vi "knob driver 3.vi"() -> ()   [LabVIEW 2015]
uses:
  Stage/Move stage command.ctl
  h-nu-ixon/knob global.vi
panel:
  out "Device numbers":i32[](array[numeric])
  out "Encoder serial numbers":i32[](array[numeric])
  in  "um per turn":dbl[](array[numeric])=[10.0, 10.0, 1.0]
  out "Knob positions":i32[](array[knob]) scale=0.0..80.0
  in  "Quit":bool
  # "x\n\ny\n\nz"
  # "x\ny\nz"
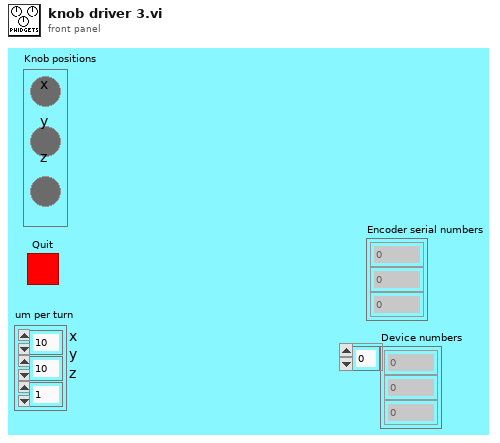
[diagram p1: front panel]
types:
  T1 = typedef "Move stage command.ctl" = cluster{"dx (um) (0 -> ignore)":ext, "dy (um) (0 -> ignore)":ext, "dz (um) (0 -> ignore)":ext, "Re-center x,y":bool, "Re-center z":bool, "x (um) (-1 -> ignore)":dbl, "y (um) (-1 -> ignore)":dbl, "z (um) (-1 -> ignore)":dbl}
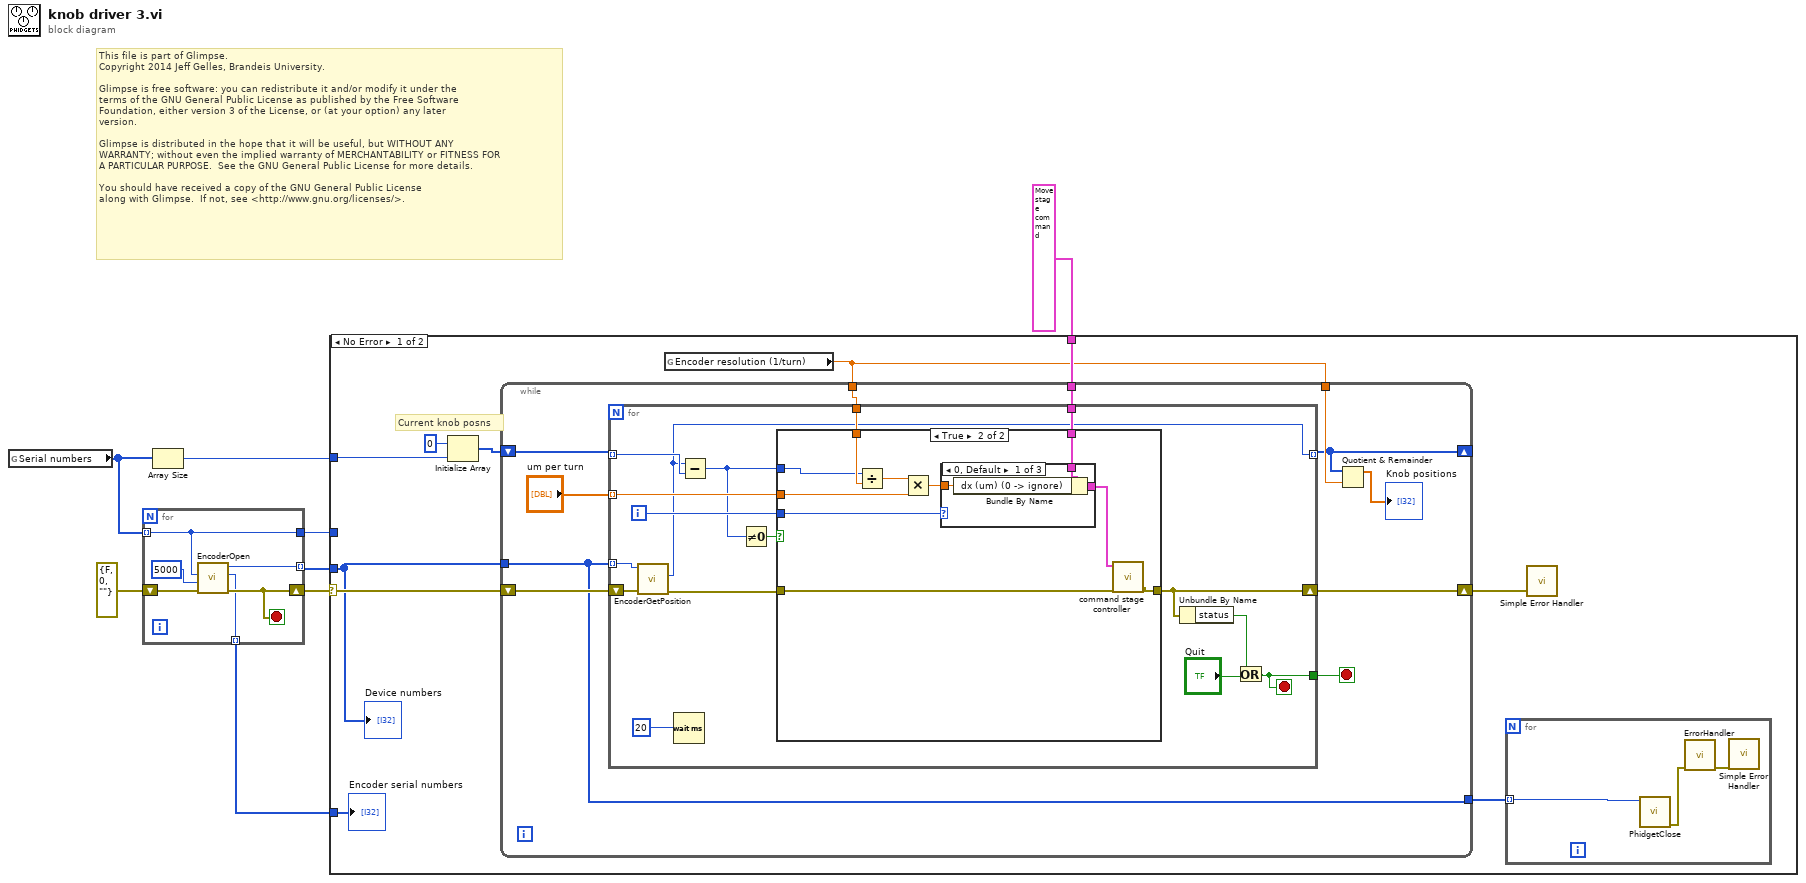
[diagram p0: block diagram]
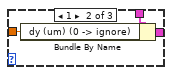
[diagram p3: hidden frame]
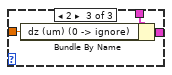
[diagram p4: hidden frame]
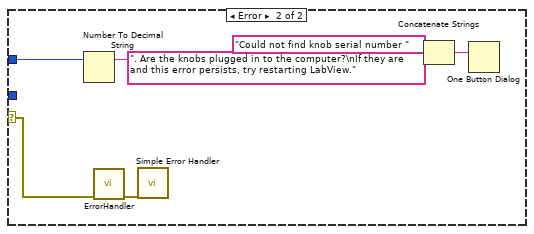
[diagram p5: hidden frame]
diagram:
  # "This file is part of Glimpse. \nCopyright 2014 Jeff Gelles, Brandeis University.    \n\nGlimpse is free software: you can redistribute it and/or modify it under the \nterms of the GNU General Public License as published by the Free Software \nFoundation, either version 3 of the License, or (at your option) any later \nversion.\n\nGlimpse is distributed in the hope that it will be useful, but WITHOUT ANY \nWARRANTY; without even the implied warranty of MERCHANTABILITY or FITNESS FOR \nA PARTICULAR PURPOSE.  See the GNU General Public License for more details.\n\nYou should have received a copy of the GNU General Public License\nalong with Glimpse.  If not, see <http://www.gnu.org/licenses/>."
  n1 = global read "knob global.vi" "Serial numbers"() -> (w4:i32[])
  n2 = for {
    tunnel: w4 -> [w11] mode=indexing
    shift-right: [w12] -> w7
    shift-left: errorcluster {"status"=FALSE, "code"=0, "source"=""} ("error in (no error)") -> [w14]
    tunnel: [w13] -> w5 mode=indexing
    tunnel: [w11] -> w6
    tunnel: [w10] -> w1 mode=indexing
    stop <- w12 stop-if-true
    n3 = call <userlib>:"EncoderOpen.vi"("error in (no error)"=w14, "milliseconds (5000)"=5000, "Serial Number (-1)"=w11) -> ("error out"=w12:errorcluster, "Serial Number Return"=w10:i32, "Device Out"=w13:i32)  [unwired: 5 in, 1 out]
  }
  n4 = Array Size(array=w4) -> (size(s)=w3:i32)
  n5 = case shown="No Error" w7 {
    selector: w7 -> [w16 w76]
    tunnel: w6 -> [_ w79]
    tunnel: w5 -> [w15 _]
    tunnel: w3 -> [w22 _]
    tunnel: T1 {"dx (um) (0 -> ignore)"=0.0, "dy (um) (0 -> ignore)"=0.0, "dz (um) (0 -> ignore)"=0.0, "Re-center x,y"=FALSE, "Re-center z"=FALSE, "x (um) (-1 -> ignore)"=-1.0, "y (um) (-1 -> ignore)"=-1.0, "z (um) (-1 -> ignore)"=-1.0} ("command") -> [w21 _]
    tunnel: w1 -> [w17 _]
    frame No Error {
      # "Current knob posns"
      n6 = Initialize Array(0 ("Position"), w22) -> (w24:i32[])
      n7 = global read "knob global.vi" "Encoder resolution (1/turn)"() -> (w20:dbl)
      n8 = while {
        shift-right: [w37] -> w19
        shift-left: w16 -> [w38]
        tunnel: w15 -> [w29]
        shift-right: [w30] -> _
        shift-left: w24 -> [w36]
        tunnel: w21 -> [w33]
        tunnel: w20 -> [w32]
        tunnel: w20 -> [w31]
        tunnel: [w29] -> w18
        stop <- w35 stop-if-true
        n9 = for {
          tunnel: w29 -> [w39] mode=indexing
          tunnel: [w47] -> w35
          shift-right: [w48] -> w37
          shift-left: w38 -> [w41]
          tunnel: [w44] -> w30 mode=indexing
          tunnel: w36 -> [w45] mode=indexing
          tunnel: "um per turn" -> [w54] mode=indexing
          tunnel: w33 -> [w53]
          tunnel: w32 -> [w51]
          i -> [w52]
          stop <- w47 stop-if-true
          n10 = call <userlib>:"EncoderGetPosition.vi"("error in (no error)"=w41, "Device In"=w39) -> ("error out"=w40:errorcluster, "Position"=w44:i32)  [unwired: 7 in, 1 out]
          n11 = Wait (ms)(milliseconds to wait=20) -> ()  [unwired: 1 out]
          n12 = Subtract(x=w44, y=w45) -> (x-y=w42:i32)
          n13 = Not Equal To 0?(x=w42) -> (x != 0?=w43:bool)
          n14 = case shown="True" w43 {
            tunnel: w54 -> [_ w65]
            tunnel: w53 -> [_ w64]
            tunnel: w52 -> [_ w63]
            tunnel: w51 -> [_ w62]
            tunnel: [w55 w61] -> w48
            tunnel: w40 -> [w55 w56]
            tunnel: w42 -> [_ w57]
            frame False {
            }
            frame True {
              n15 = Divide(x=w57, y=w62) -> (x/y=w58:dbl)
              n16 = Multiply(x=w58, y=w65) -> (x*y=w59:dbl)
              n17 = case shown="0, Default" w63 {
                tunnel: w64 -> [w68 w71 w74]
                tunnel: [w67 w70 w73] -> w60
                tunnel: w59 -> [w66 w69 w72]
                frame 0, Default {
                  n18 = Bundle By Name(cluster=w68, "dx (um) (0 -> ignore)"=w66) -> (w67:T1)
                }
                frame 1 {
                  n19 = Bundle By Name(cluster=w71, "dy (um) (0 -> ignore)"=w69) -> (w70:T1)
                }
                frame 2 {
                  n20 = Bundle By Name(cluster=w74, "dz (um) (0 -> ignore)"=w72) -> (w73:T1)
                }
              }
              n21 = call "command stage controller.vi"("command"=w60, "error in (no error)"=w56) -> ("error out"=w61:errorcluster)  [unwired: 6 in]
            }
          }
          n22 = Unbundle By Name(w48) -> ("status"=w49:bool)
          n23 = Or(x=w49, y="Quit") -> (x .or. y?=w47:bool)
        }
        n24 = Quotient & Remainder(x=w30, y=w31) -> (x-y*floor(x/y)=→"Knob positions":dbl[])  [unwired: 1 out]
      }
      n25 = for {
        tunnel: w18 -> [w25] mode=indexing
        n26 = call <userlib>:"PhidgetClose.vi"("Device In"=w25) -> ("error out"=w26:errorcluster)  [unwired: 10 in]
        n27 = call <userlib>:"ErrorHandler.vi"("error in"=w26) -> ("error out"=w27:errorcluster)  [unwired: 9 in, 1 out]
        n28 = call <vilib>:"Simple Error Handler.vi"("error in (no error)"=w27) -> ()  [unwired: 4 in, 5 out]
      }
      n29 = call <vilib>:"Simple Error Handler.vi"("error in (no error)"=w19) -> ()  [unwired: 4 in, 5 out]
      "Encoder serial numbers" <- w17
      "Device numbers" <- w15
    }
    frame Error {
      n30 = Number To Decimal String(number=w79) -> (decimal integer string=w78:string)  [unwired: 1 in]
      n31 = call <userlib>:"ErrorHandler.vi"("error in"=w76) -> ("error out"=w75:errorcluster)  [unwired: 9 in, 1 out]
      n32 = call <vilib>:"Simple Error Handler.vi"("error in (no error)"=w75) -> ()  [unwired: 4 in, 5 out]
      n33 = Concatenate Strings("Could not find knob serial number " ("string"), w78, ". Are the knobs plugged in to the computer?\nIf they are and this error persists, try restarting LabView." ("string")) -> (w81:string)
      n34 = One Button Dialog(message=w81) -> ()  [unwired: 1 in, 1 out]
    }
  }
